vi "Get Routine Object.vi"(7 "Settings":T2=enum."Custom", 8 "error in (no error)":errorcluster, 10 "6 Inch":bool, 11 "Routine":T1=enum."Secure Syringe") -> (0 "error out":errorcluster, 3 "Routine out":refnum<class "Routine.lvclass">)   [LabVIEW 2016, in "Routine.lvclass"]
uses:
  Routine.lvclass
  Settings.ctl
  Routine Enum.ctl
  Dispense/Iterative Dispense/Glue Step Enum.ctl
  Dispense/Iterative Dispense/8 inch/8 Inch Iterative Dispense.lvclass
  D:/UCSB-Gantry_ms/UCSB-Gantry 0518/V5/Classes/Routine/Dispense/Iterative Dispense/Iterative Dispense.lvclass
  Dispense/Iterative Dispense/Iterative Dispense.lvclass/Iterative Dispense.ctl
  Pick and Place/Pick and Place.lvclass
  D:/UCSB-Gantry_ms/UCSB-Gantry 0518/V5/Classes/Routine/Routine.lvclass
  Pick and Place/Pick and Place Type.ctl
  Pick and Place/Pick and Place.lvclass/Pick and Place.ctl
  Secure Syringe/SecureRelease Syringe.lvclass
  Secure Syringe/SecureRelease Syringe.lvclass/SecureRelease Syringe.ctl
  Dispense/CAD Dispense/8 Inch CAD Dispense.lvclass
  D:/UCSB-Gantry_ms/UCSB-Gantry 0518/V5/Classes/Routine/Dispense/CAD Dispense/CAD Dispense.lvclass
  Dispense/CAD Dispense2/CAD Dispense2.lvclass
  Dispense/Iterative Dispense/Write Glue Step Enum.vi
  Pick and Place/Write Pick and Place Type.vi
  Secure Syringe/Write Type.vi
  Dispense/Iterative Dispense/Iterative Dispense.lvclass
  Dispense/CAD Dispense/CAD Dispense.lvclass
  Dispense/Iterative Dispense/6 inch/6 Inch Iterative Dispense.lvclass
  Dispense/CAD Dispense/6 inch CAD Dispense.lvclass
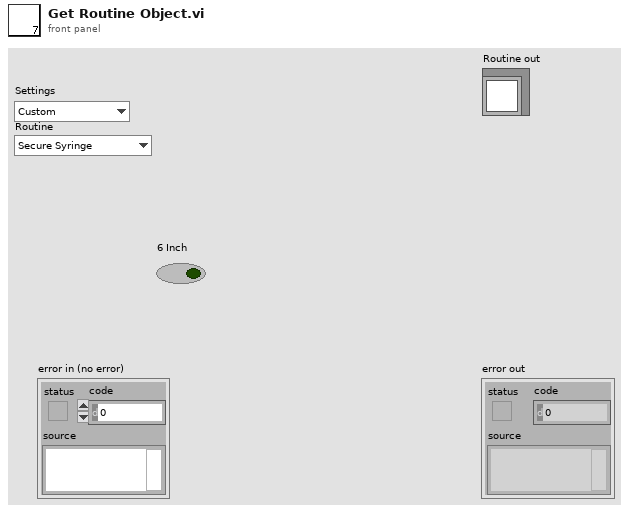
[diagram p1: front panel]
types:
  T1 = typedef "Routine.lvclass/Routine Enum.ctl" = enum16{"Primary Pick Up", "Pick Up All", "Put Down Secondary", "Put Down All", "Release Syringe", "Secondary Pick Up", "Secure Syringe", "Dispense on Plate", "Dispense on Kapton", "Dispense on Sensor", "Dispense on Sensor2"}
  T2 = typedef "Routine.lvclass/Settings.ctl" = enum16{"Default", "Custom"}
  T3 = typedef "Pick and Place.lvclass/Pick and Place Type.ctl" = enum16{"Primary Pick Up", "Secondary Pick Up", "Put Down All", "Pick Up All", "Put Down Secondary"}
  T4 = typedef "Iterative Dispense.lvclass/Glue Step Enum.ctl" = enum16{"Baseplate to Kapton", "Kapton to Sensor"}
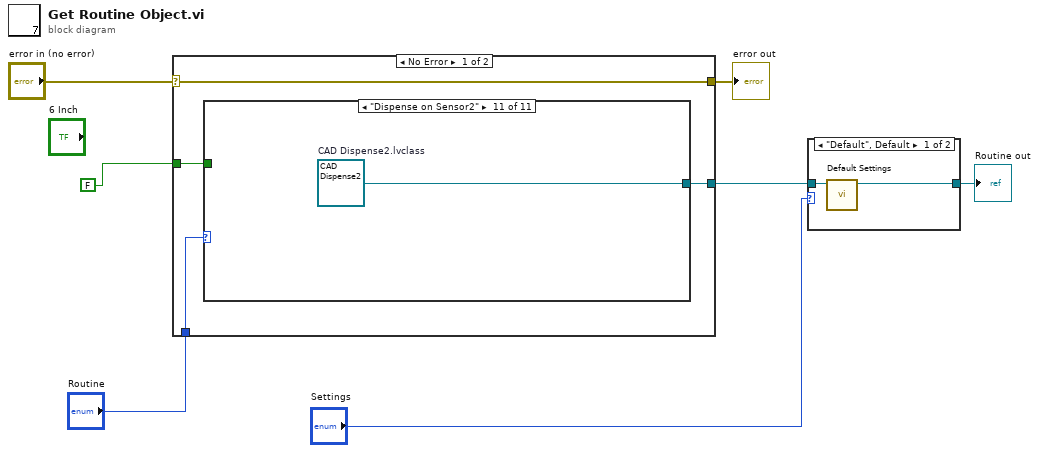
[diagram p0: block diagram]
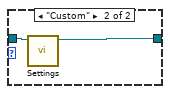
[diagram p2: hidden frame]
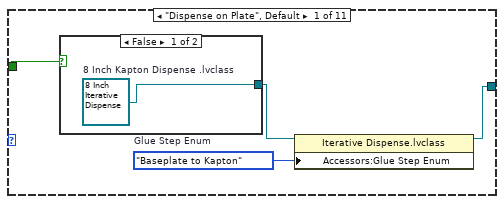
[diagram p3: hidden frame]
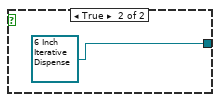
[diagram p4: hidden frame]
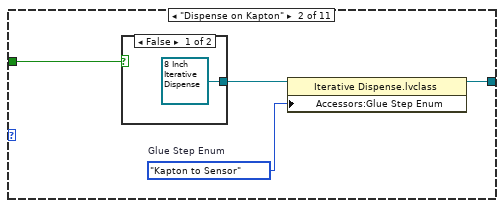
[diagram p5: hidden frame]
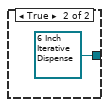
[diagram p6: hidden frame]
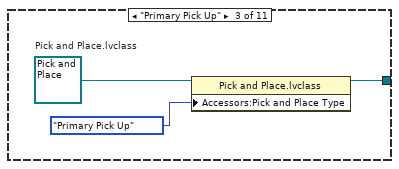
[diagram p7: hidden frame]
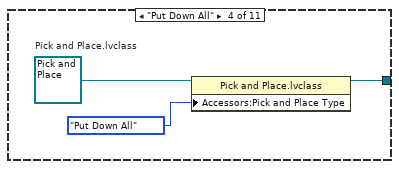
[diagram p8: hidden frame]
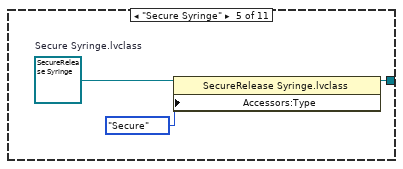
[diagram p9: hidden frame]
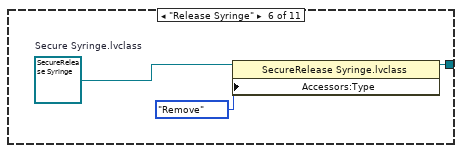
[diagram p10: hidden frame]
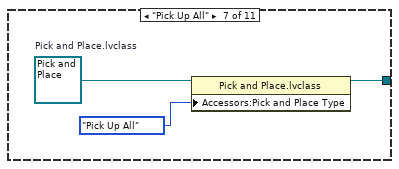
[diagram p11: hidden frame]
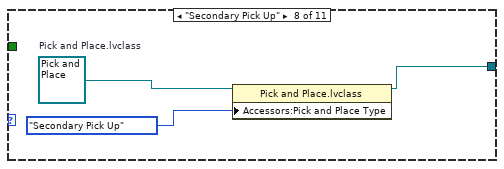
[diagram p12: hidden frame]
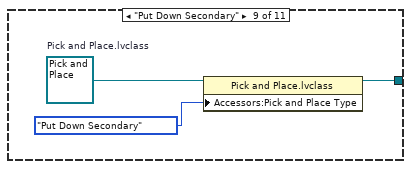
[diagram p13: hidden frame]
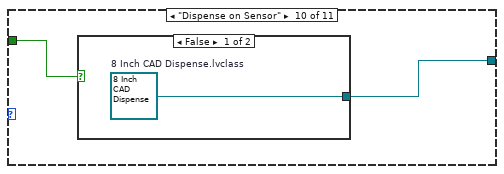
[diagram p14: hidden frame]
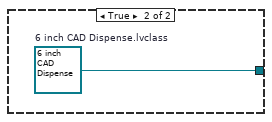
[diagram p15: hidden frame]
diagram:
  n1 = case shown="No Error" "error in (no error)" {
    selector: "error in (no error)" -> [w11 w50]
    tunnel: [w11 w50] -> w6
    tunnel: [w10 _] -> w5
    tunnel: FALSE -> [w9 _]
    tunnel: "Routine" -> [w8 _]
    frame No Error {
      n2 = case shown="\"Dispense on Sensor2\"" w8 {
        tunnel: [w15 w21 w25 w28 w30 w33 w36 w39 w42 w46 w49] -> w10
        tunnel: w9 -> [w13 w19 _ _ _ _ _ _ _ w45 _]
        frame "Dispense on Plate", Default {
          w14 = Glue_Step_Enum."Baseplate to Kapton"  # Glue Step Enum
          n3 = case shown="False" w13 {
            tunnel: [w16 refnum<class "6 Inch Iterative Dispense.lvclass"> refnum ("6 Inch Kapton Dispense.lvclass")] -> w12
            frame False {
              w16 = refnum<class "8 Inch Iterative Dispense.lvclass"> refnum  # 8 Inch Kapton Dispense .lvclass
            }
            frame True {
            }
          }
          n4 = property class="Iterative Dispense.lvclass"(reference=w12, "Accessors:Glue Step Enum"=w14) -> (reference out=w15:refnum<class "Iterative Dispense.lvclass">)  [unwired: 1 in, 1 out]
        }
        frame "Dispense on Kapton" {
          w20 = Glue_Step_Enum."Kapton to Sensor"  # Glue Step Enum
          n5 = case shown="False" w19 {
            tunnel: [refnum<class "8 Inch Iterative Dispense.lvclass"> refnum ("8 Inch Kapton Dispense .lvclass") refnum<class "6 Inch Iterative Dispense.lvclass"> refnum ("6 Inch Kapton Dispense.lvclass")] -> w18
            frame False {
            }
            frame True {
            }
          }
          n6 = property class="Iterative Dispense.lvclass"(reference=w18, "Accessors:Glue Step Enum"=w20) -> (reference out=w21:refnum<class "Iterative Dispense.lvclass">)  [unwired: 1 in, 1 out]
        }
        frame "Primary Pick Up" {
          w26 = refnum<class "Pick and Place.lvclass"> refnum  # Pick and Place.lvclass
          n7 = property class="Pick and Place.lvclass"(reference=w26, "Accessors:Pick and Place Type"=Pick_and_Place_Type."Primary Pick Up" ("Pick and Place Type")) -> (reference out=w25:refnum<class "Pick and Place.lvclass">)  [unwired: 1 in, 1 out]
        }
        frame "Put Down All" {
          w29 = refnum<class "Pick and Place.lvclass"> refnum  # Pick and Place.lvclass
          n8 = property class="Pick and Place.lvclass"(reference=w29, "Accessors:Pick and Place Type"=Pick_and_Place_Type."Put Down All" ("Pick and Place Type")) -> (reference out=w28:refnum<class "Pick and Place.lvclass">)  [unwired: 1 in, 1 out]
        }
        frame "Secure Syringe" {
          w32 = refnum<class "SecureRelease Syringe.lvclass"> refnum  # Secure Syringe.lvclass
          n9 = property class="SecureRelease Syringe.lvclass"(reference=w32, "Accessors:Type"=enum16{"Secure", "Remove"}."Secure" ("Type")) -> (reference out=w30:refnum<class "SecureRelease Syringe.lvclass">)  [unwired: 1 in, 1 out]
        }
        frame "Release Syringe" {
          w35 = refnum<class "SecureRelease Syringe.lvclass"> refnum  # Secure Syringe.lvclass
          n10 = property class="SecureRelease Syringe.lvclass"(reference=w35, "Accessors:Type"=enum16{"Secure", "Remove"}."Remove" ("Type")) -> (reference out=w33:refnum<class "SecureRelease Syringe.lvclass">)  [unwired: 1 in, 1 out]
        }
        frame "Pick Up All" {
          w38 = refnum<class "Pick and Place.lvclass"> refnum  # Pick and Place.lvclass
          n11 = property class="Pick and Place.lvclass"(reference=w38, "Accessors:Pick and Place Type"=Pick_and_Place_Type."Pick Up All" ("Pick and Place Type")) -> (reference out=w36:refnum<class "Pick and Place.lvclass">)  [unwired: 1 in, 1 out]
        }
        frame "Secondary Pick Up" {
          w41 = refnum<class "Pick and Place.lvclass"> refnum  # Pick and Place.lvclass
          n12 = property class="Pick and Place.lvclass"(reference=w41, "Accessors:Pick and Place Type"=Pick_and_Place_Type."Secondary Pick Up" ("Pick and Place Type")) -> (reference out=w39:refnum<class "Pick and Place.lvclass">)  [unwired: 1 in, 1 out]
        }
        frame "Put Down Secondary" {
          w44 = refnum<class "Pick and Place.lvclass"> refnum  # Pick and Place.lvclass
          n13 = property class="Pick and Place.lvclass"(reference=w44, "Accessors:Pick and Place Type"=Pick_and_Place_Type."Put Down Secondary" ("Pick and Place Type")) -> (reference out=w42:refnum<class "Pick and Place.lvclass">)  [unwired: 1 in, 1 out]
        }
        frame "Dispense on Sensor" {
          n14 = case shown="False" w45 {
            tunnel: [w47 w48] -> w46
            frame False {
              w47 = refnum<class "8 Inch CAD Dispense.lvclass"> refnum  # 8 Inch CAD Dispense.lvclass
            }
            frame True {
              w48 = refnum<class "6 inch CAD Dispense.lvclass"> refnum  # 6 inch CAD Dispense.lvclass
            }
          }
        }
        frame "Dispense on Sensor2" {
          w49 = refnum<class "CAD Dispense2.lvclass"> refnum  # CAD Dispense2.lvclass
        }
      }
    }
    frame Error {
    }
  }
  "error out" <- w6
  n15 = case shown="\"Default\", Default" "Settings" {
    tunnel: w5 -> [w52 w54]
    tunnel: [w51 w53] -> w4
    frame "Default", Default {
      n16 = call-dynamic "Default Settings.vi"("Routine in"=w52) -> ("Routine out"=w51:refnum<class "Routine.lvclass">)  [unwired: 9 in, 1 out]
    }
    frame "Custom" {
      n17 = call-dynamic "Settings.vi"("Routine in"=w54) -> ("Routine out"=w53:refnum<class "Routine.lvclass">)  [unwired: 9 in, 1 out]
    }
  }
  "Routine out" <- w4
